vi "3. 绘制：管道分布 图.vi"(2 "放大倍数":i32, 3 "坐标原点 重新选定后 的 一维数组":dbl[](array[numeric]), 4 "color(black)输入":u32(colorbox)=8816506 caption="管道颜色") -> (0 "管道分布":picture)   [LabVIEW 2018]
panel:
  in  "初始白图":picture
  in  "fill?(F)输入":bool=TRUE caption="管道：填充？(F)"
  in  "pen输入":T1={"Width"=1, "Style"=enum."Solid"} caption="管道画笔"
  out "管道":picture
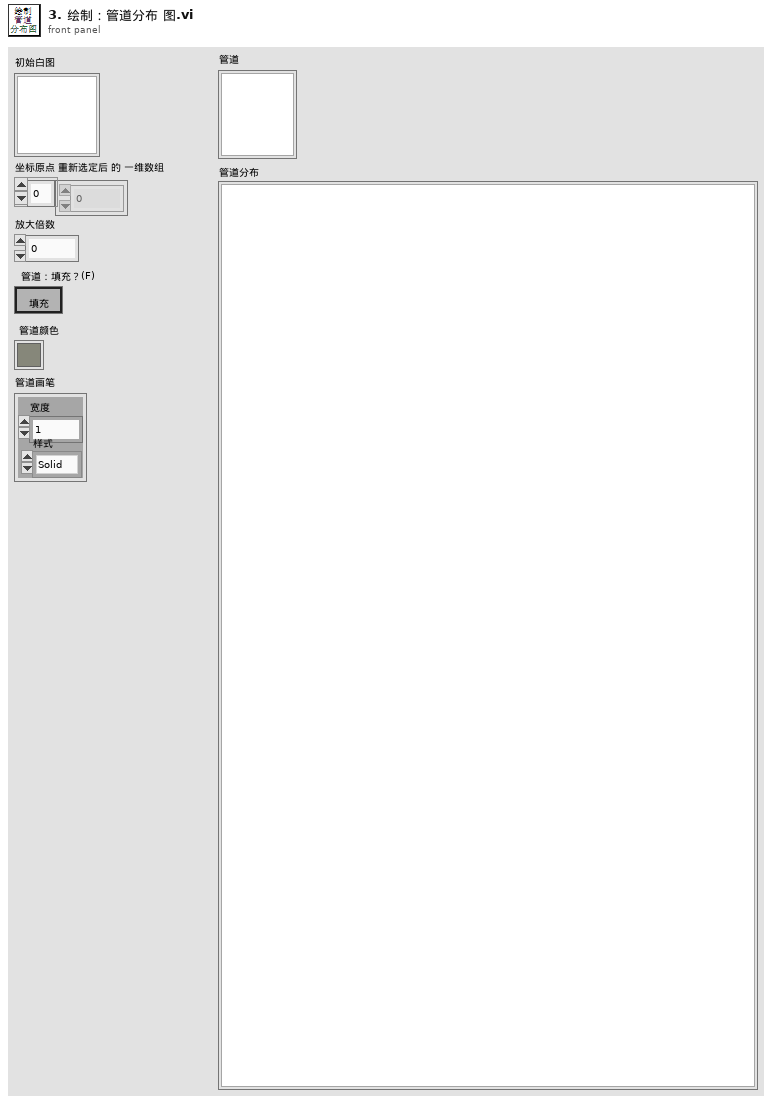
[diagram p1: front panel]
types:
  T1 = cluster{"Width":i16, "Style":enum32{"Solid", "Dash", "Dot", "DashDot", "DashDotDot"}}
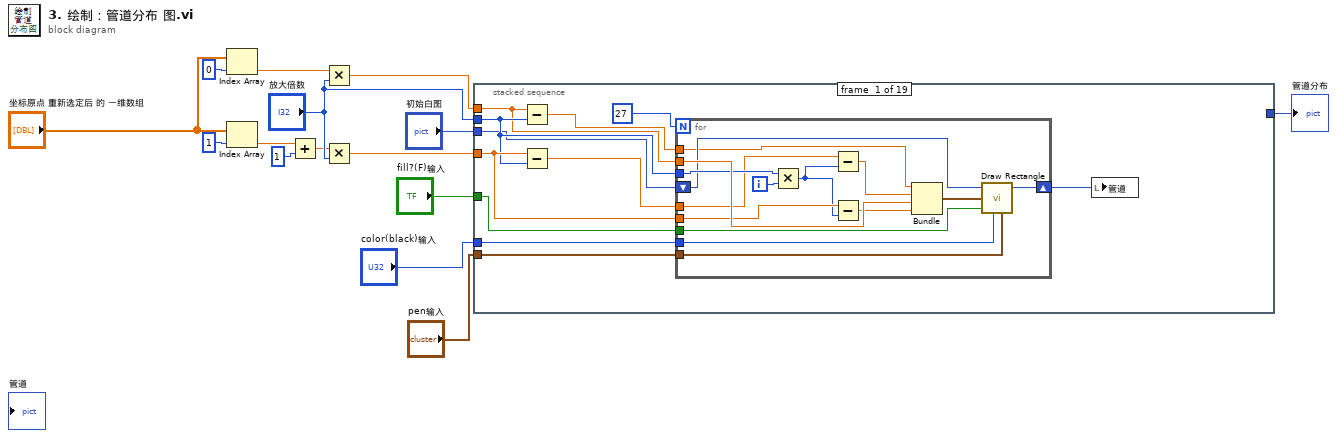
[diagram p0: block diagram]
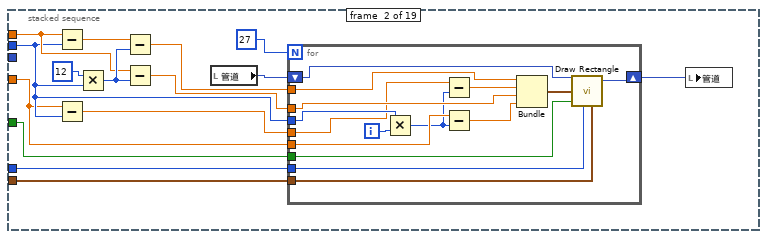
[diagram p2: hidden frame]
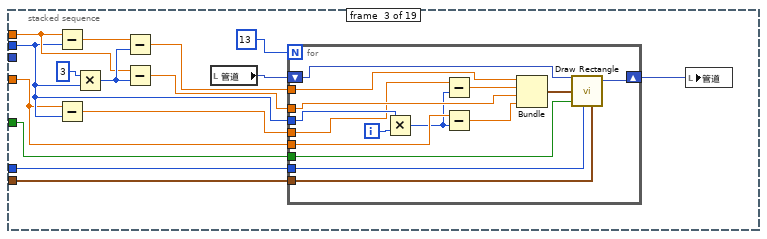
[diagram p3: hidden frame]
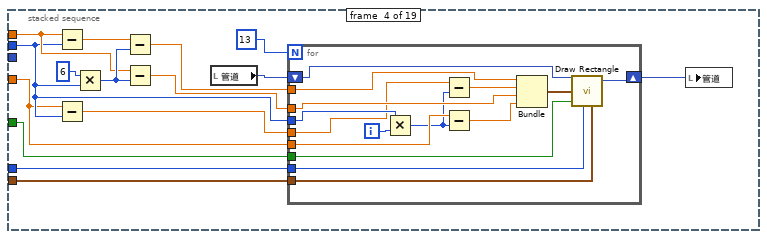
[diagram p4: hidden frame]
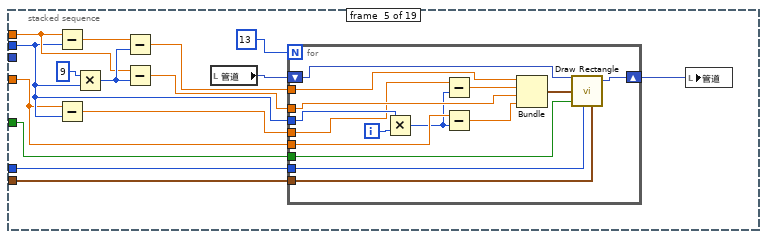
[diagram p5: hidden frame]
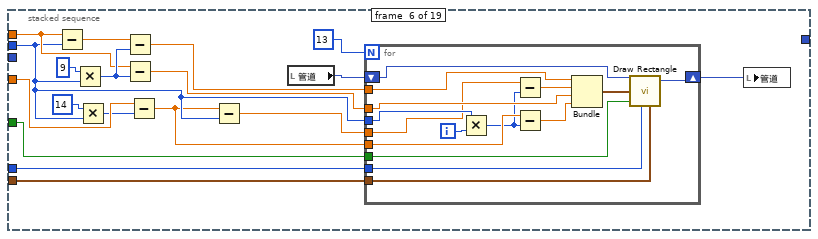
[diagram p6: hidden frame]
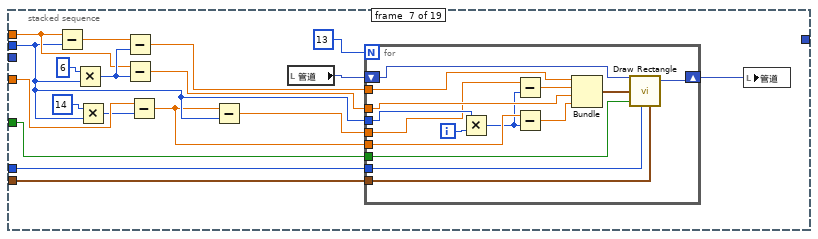
[diagram p7: hidden frame]
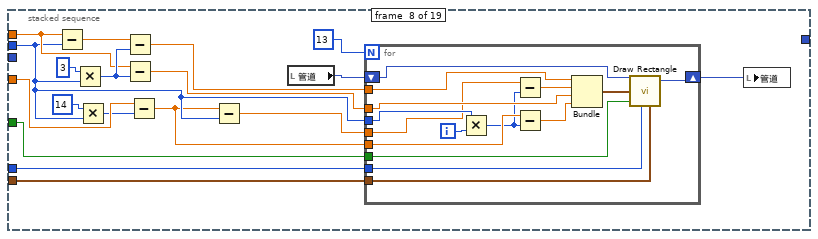
[diagram p8: hidden frame]
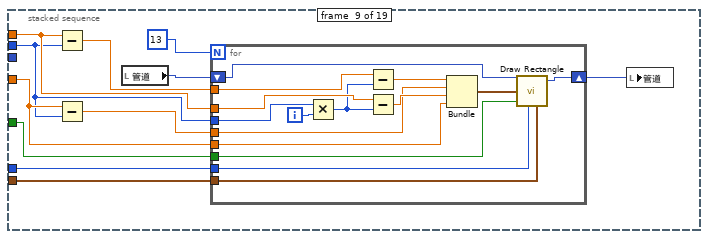
[diagram p9: hidden frame]
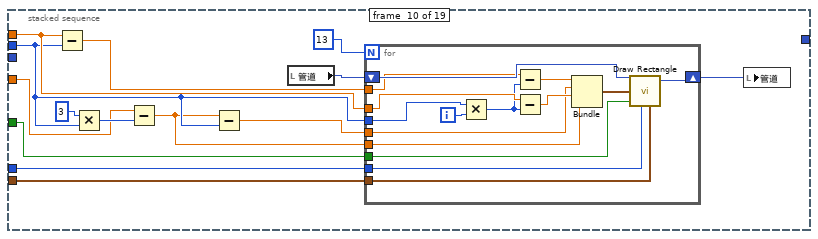
[diagram p10: hidden frame]
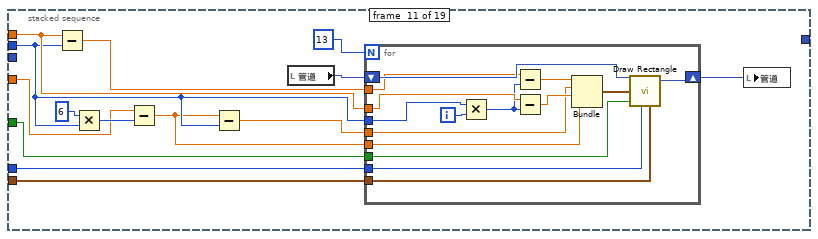
[diagram p11: hidden frame]
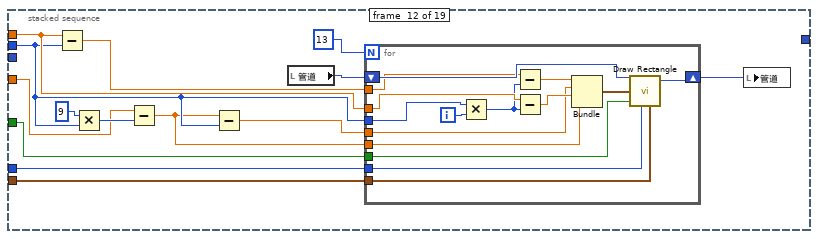
[diagram p12: hidden frame]
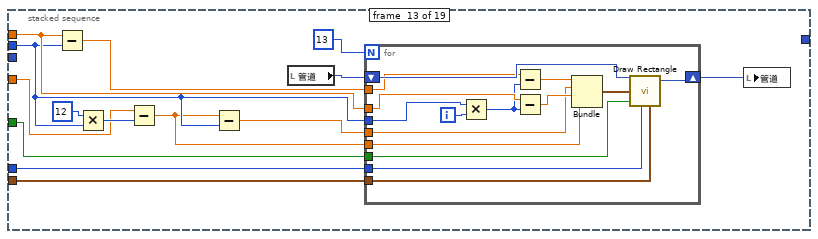
[diagram p13: hidden frame]
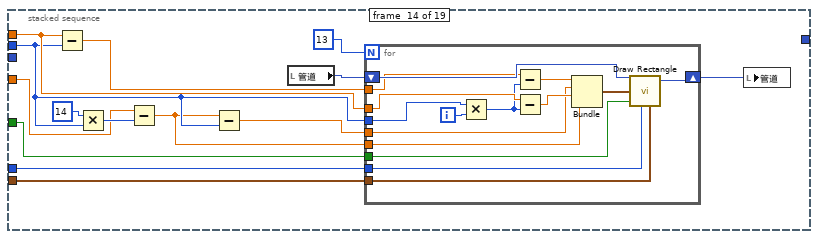
[diagram p14: hidden frame]
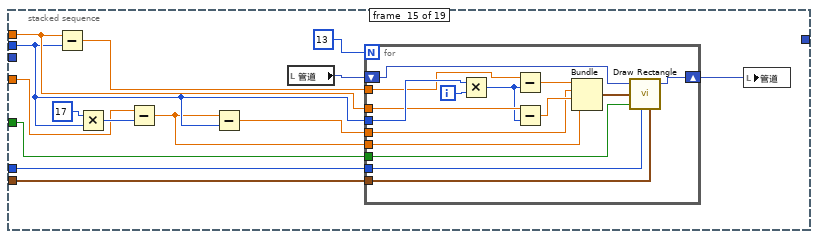
[diagram p15: hidden frame]
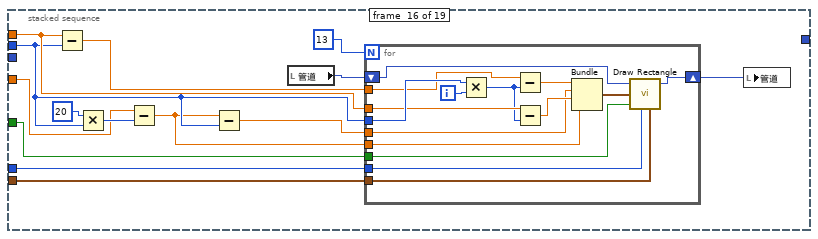
[diagram p16: hidden frame]
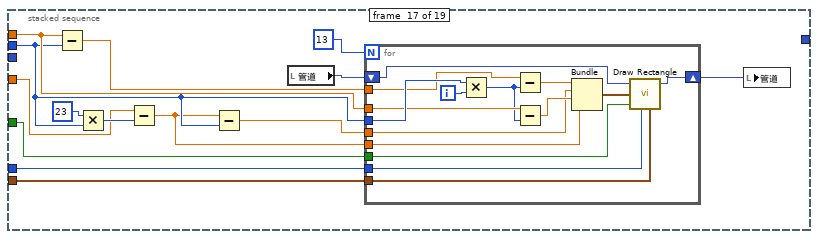
[diagram p17: hidden frame]
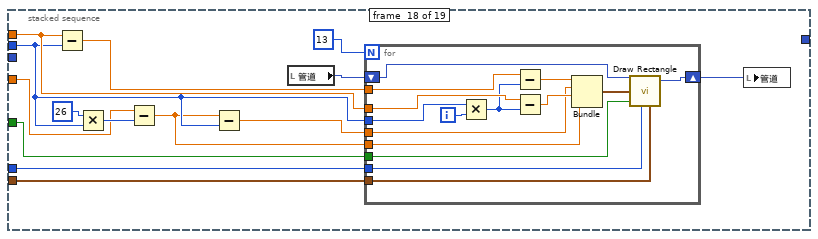
[diagram p18: hidden frame]
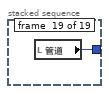
[diagram p19: hidden frame]
diagram:
  n1 = Index Array(array="坐标原点 重新选定后 的 一维数组", index=0) -> (element=w6:dbl)
  n2 = Index Array(array="坐标原点 重新选定后 的 一维数组", index=1) -> (element=w3:dbl)
  n3 = Add(x=w3, y=1) -> (x+y=w5:dbl)
  n4 = Multiply(x=w6, y="放大倍数") -> (x*y=w11:dbl)
  n5 = Multiply(x=w5, y="放大倍数") -> (x*y=w10:dbl)
  n6 = stacked-sequence {
    tunnel: "pen输入" -> [w25 w55 w85 w115 w145 w178 w211 w244 w270 w299 w328 w357 w386 w415 w444 w473 w502 w531 _]
    tunnel: "color(black)输入" -> [w24 w54 w84 w114 w144 w177 w210 w243 w269 w298 w327 w356 w385 w414 w443 w472 w501 w530 _]
    tunnel: "fill?(F)输入" -> [w23 w53 w83 w113 w143 w176 w209 w242 w268 w297 w326 w355 w384 w413 w442 w471 w500 w529 _]
    tunnel: w10 -> [w20 w44 w74 w104 w134 w165 w198 w231 w265 w290 w319 w348 w377 w406 w435 w464 w493 w522 _]
    tunnel: "放大倍数" -> [w19 w45 w75 w105 w135 w167 w200 w233 w264 w293 w322 w351 w380 w409 w438 w467 w496 w525 _]
    tunnel: w11 -> [w18 w46 w76 w106 w136 w169 w202 w235 w267 w296 w325 w354 w383 w412 w441 w470 w499 w528 _]
    tunnel: "初始白图" -> [w16 _ _ _ _ _ _ _ _ _ _ _ _ _ _ _ _ _ _]
    tunnel: [_ _ _ _ _ _ _ _ _ _ _ _ _ _ _ _ _ _ w548] -> w13
    frame #0 {
      n7 = Subtract(x=w18, y=w19) -> (x-y=w22:dbl)
      n8 = Subtract(x=w20, y=w19) -> (x-y=w21:dbl)
      n9 = for {
        N: 27 -> [_]
        shift-right: [w41] -> w17
        shift-left: w16 -> [w35]
        tunnel: w20 -> [w38]
        tunnel: w18 -> [w40]
        tunnel: w19 -> [w39]
        tunnel: w25 -> [w33]
        tunnel: w24 -> [w32]
        tunnel: w23 -> [w31]
        tunnel: w21 -> [w29]
        tunnel: w22 -> [w28]
        i -> [w30]
        n10 = Multiply(x=w39, y=w30) -> (x*y=w27:i32)
        n11 = Subtract(x=w29, y=w27) -> (x-y=w36:dbl)
        n12 = Subtract(x=w38, y=w27) -> (x-y=w37:dbl)
        n13 = Bundle(w28, w36, w40, w37) -> (w34:cluster{dbl, dbl, dbl, dbl})  [unwired: 1 in]
        n14 = call <vilib>:"Draw Rectangle.vi"("picture"=w35, "rect"=w34, "fill?(F)"=w31, "color(black)"=w32, "pen"=w33) -> ("new picture"=w41:picture)  [unwired: 4 in]
      }
      n15 = local write "管道"(w17) -> ()
    }
    frame #1 {
      n16 = Subtract(x=w46, y=w45) -> (x-y=w47:dbl)
      n17 = Subtract(x=w44, y=w45) -> (x-y=w51:dbl)
      n18 = Multiply(x=12, y=w45) -> (x*y=w48:i32)
      n19 = Subtract(x=w47, y=w48) -> (x-y=w52:dbl)
      n20 = Subtract(x=w46, y=w48) -> (x-y=w49:dbl)
      n21 = local read "管道"() -> (w42:picture)
      n22 = for {
        N: 27 -> [_]
        shift-right: [w71] -> w43
        shift-left: w42 -> [w66]
        tunnel: w44 -> [w68]
        tunnel: w49 -> [w70]
        tunnel: w45 -> [w69]
        tunnel: w55 -> [w64]
        tunnel: w54 -> [w63]
        tunnel: w53 -> [w62]
        tunnel: w51 -> [w60]
        tunnel: w52 -> [w58]
        i -> [w61]
        n23 = Multiply(x=w69, y=w61) -> (x*y=w59:i32)
        n24 = Subtract(x=w60, y=w59) -> (x-y=w57:dbl)
        n25 = Subtract(x=w68, y=w59) -> (x-y=w67:dbl)
        n26 = Bundle(w58, w57, w70, w67) -> (w65:cluster{dbl, dbl, dbl, dbl})  [unwired: 1 in]
        n27 = call <vilib>:"Draw Rectangle.vi"("picture"=w66, "rect"=w65, "fill?(F)"=w62, "color(black)"=w63, "pen"=w64) -> ("new picture"=w71:picture)  [unwired: 4 in]
      }
      n28 = local write "管道"(w43) -> ()
    }
    frame #2 {
      n29 = Subtract(x=w76, y=w75) -> (x-y=w77:dbl)
      n30 = Subtract(x=w74, y=w75) -> (x-y=w81:dbl)
      n31 = Multiply(x=3, y=w75) -> (x*y=w78:i32)
      n32 = Subtract(x=w77, y=w78) -> (x-y=w82:dbl)
      n33 = Subtract(x=w76, y=w78) -> (x-y=w79:dbl)
      n34 = local read "管道"() -> (w72:picture)
      n35 = for {
        N: 13 -> [_]
        shift-right: [w101] -> w73
        shift-left: w72 -> [w96]
        tunnel: w74 -> [w98]
        tunnel: w79 -> [w100]
        tunnel: w75 -> [w99]
        tunnel: w85 -> [w94]
        tunnel: w84 -> [w93]
        tunnel: w83 -> [w92]
        tunnel: w81 -> [w90]
        tunnel: w82 -> [w88]
        i -> [w91]
        n36 = Multiply(x=w99, y=w91) -> (x*y=w89:i32)
        n37 = Subtract(x=w90, y=w89) -> (x-y=w87:dbl)
        n38 = Subtract(x=w98, y=w89) -> (x-y=w97:dbl)
        n39 = Bundle(w88, w87, w100, w97) -> (w95:cluster{dbl, dbl, dbl, dbl})  [unwired: 1 in]
        n40 = call <vilib>:"Draw Rectangle.vi"("picture"=w96, "rect"=w95, "fill?(F)"=w92, "color(black)"=w93, "pen"=w94) -> ("new picture"=w101:picture)  [unwired: 4 in]
      }
      n41 = local write "管道"(w73) -> ()
    }
    frame #3 {
      n42 = Subtract(x=w106, y=w105) -> (x-y=w107:dbl)
      n43 = Subtract(x=w104, y=w105) -> (x-y=w111:dbl)
      n44 = Multiply(x=6, y=w105) -> (x*y=w108:i32)
      n45 = Subtract(x=w107, y=w108) -> (x-y=w112:dbl)
      n46 = Subtract(x=w106, y=w108) -> (x-y=w109:dbl)
      n47 = local read "管道"() -> (w102:picture)
      n48 = for {
        N: 13 -> [_]
        shift-right: [w131] -> w103
        shift-left: w102 -> [w126]
        tunnel: w104 -> [w128]
        tunnel: w109 -> [w130]
        tunnel: w105 -> [w129]
        tunnel: w115 -> [w124]
        tunnel: w114 -> [w123]
        tunnel: w113 -> [w122]
        tunnel: w111 -> [w120]
        tunnel: w112 -> [w118]
        i -> [w121]
        n49 = Multiply(x=w129, y=w121) -> (x*y=w119:i32)
        n50 = Subtract(x=w120, y=w119) -> (x-y=w117:dbl)
        n51 = Subtract(x=w128, y=w119) -> (x-y=w127:dbl)
        n52 = Bundle(w118, w117, w130, w127) -> (w125:cluster{dbl, dbl, dbl, dbl})  [unwired: 1 in]
        n53 = call <vilib>:"Draw Rectangle.vi"("picture"=w126, "rect"=w125, "fill?(F)"=w122, "color(black)"=w123, "pen"=w124) -> ("new picture"=w131:picture)  [unwired: 4 in]
      }
      n54 = local write "管道"(w103) -> ()
    }
    frame #4 {
      n55 = Subtract(x=w136, y=w135) -> (x-y=w137:dbl)
      n56 = Subtract(x=w134, y=w135) -> (x-y=w141:dbl)
      n57 = Multiply(x=9, y=w135) -> (x*y=w138:i32)
      n58 = Subtract(x=w137, y=w138) -> (x-y=w142:dbl)
      n59 = Subtract(x=w136, y=w138) -> (x-y=w139:dbl)
      n60 = local read "管道"() -> (w132:picture)
      n61 = for {
        N: 13 -> [_]
        shift-right: [w161] -> w133
        shift-left: w132 -> [w156]
        tunnel: w134 -> [w158]
        tunnel: w139 -> [w160]
        tunnel: w135 -> [w159]
        tunnel: w145 -> [w154]
        tunnel: w144 -> [w153]
        tunnel: w143 -> [w152]
        tunnel: w141 -> [w150]
        tunnel: w142 -> [w148]
        i -> [w151]
        n62 = Multiply(x=w159, y=w151) -> (x*y=w149:i32)
        n63 = Subtract(x=w150, y=w149) -> (x-y=w147:dbl)
        n64 = Subtract(x=w158, y=w149) -> (x-y=w157:dbl)
        n65 = Bundle(w148, w147, w160, w157) -> (w155:cluster{dbl, dbl, dbl, dbl})  [unwired: 1 in]
        n66 = call <vilib>:"Draw Rectangle.vi"("picture"=w156, "rect"=w155, "fill?(F)"=w152, "color(black)"=w153, "pen"=w154) -> ("new picture"=w161:picture)  [unwired: 4 in]
      }
      n67 = local write "管道"(w133) -> ()
    }
    frame #5 {
      n68 = Subtract(x=w169, y=w167) -> (x-y=w170:dbl)
      n69 = Multiply(x=9, y=w167) -> (x*y=w171:i32)
      n70 = Multiply(x=14, y=w167) -> (x*y=w164:i32)
      n71 = Subtract(x=w170, y=w171) -> (x-y=w175:dbl)
      n72 = Subtract(x=w169, y=w171) -> (x-y=w172:dbl)
      n73 = Subtract(x=w165, y=w164) -> (x-y=w166:dbl)
      n74 = Subtract(x=w166, y=w167) -> (x-y=w174:dbl)
      n75 = local read "管道"() -> (w162:picture)
      n76 = for {
        N: 13 -> [_]
        shift-right: [w194] -> w163
        shift-left: w162 -> [w189]
        tunnel: w166 -> [w191]
        tunnel: w172 -> [w193]
        tunnel: w167 -> [w192]
        tunnel: w178 -> [w187]
        tunnel: w177 -> [w186]
        tunnel: w176 -> [w185]
        tunnel: w174 -> [w183]
        tunnel: w175 -> [w181]
        i -> [w184]
        n77 = Multiply(x=w192, y=w184) -> (x*y=w182:i32)
        n78 = Subtract(x=w183, y=w182) -> (x-y=w180:dbl)
        n79 = Subtract(x=w191, y=w182) -> (x-y=w190:dbl)
        n80 = Bundle(w181, w180, w193, w190) -> (w188:cluster{dbl, dbl, dbl, dbl})  [unwired: 1 in]
        n81 = call <vilib>:"Draw Rectangle.vi"("picture"=w189, "rect"=w188, "fill?(F)"=w185, "color(black)"=w186, "pen"=w187) -> ("new picture"=w194:picture)  [unwired: 4 in]
      }
      n82 = local write "管道"(w163) -> ()
    }
    frame #6 {
      n83 = Subtract(x=w202, y=w200) -> (x-y=w203:dbl)
      n84 = Multiply(x=6, y=w200) -> (x*y=w204:i32)
      n85 = Multiply(x=14, y=w200) -> (x*y=w197:i32)
      n86 = Subtract(x=w203, y=w204) -> (x-y=w208:dbl)
      n87 = Subtract(x=w202, y=w204) -> (x-y=w205:dbl)
      n88 = Subtract(x=w198, y=w197) -> (x-y=w199:dbl)
      n89 = Subtract(x=w199, y=w200) -> (x-y=w207:dbl)
      n90 = local read "管道"() -> (w195:picture)
      n91 = for {
        N: 13 -> [_]
        shift-right: [w227] -> w196
        shift-left: w195 -> [w222]
        tunnel: w199 -> [w224]
        tunnel: w205 -> [w226]
        tunnel: w200 -> [w225]
        tunnel: w211 -> [w220]
        tunnel: w210 -> [w219]
        tunnel: w209 -> [w218]
        tunnel: w207 -> [w216]
        tunnel: w208 -> [w214]
        i -> [w217]
        n92 = Multiply(x=w225, y=w217) -> (x*y=w215:i32)
        n93 = Subtract(x=w216, y=w215) -> (x-y=w213:dbl)
        n94 = Subtract(x=w224, y=w215) -> (x-y=w223:dbl)
        n95 = Bundle(w214, w213, w226, w223) -> (w221:cluster{dbl, dbl, dbl, dbl})  [unwired: 1 in]
        n96 = call <vilib>:"Draw Rectangle.vi"("picture"=w222, "rect"=w221, "fill?(F)"=w218, "color(black)"=w219, "pen"=w220) -> ("new picture"=w227:picture)  [unwired: 4 in]
      }
      n97 = local write "管道"(w196) -> ()
    }
    frame #7 {
      n98 = Subtract(x=w235, y=w233) -> (x-y=w236:dbl)
      n99 = Multiply(x=3, y=w233) -> (x*y=w237:i32)
      n100 = Multiply(x=14, y=w233) -> (x*y=w230:i32)
      n101 = Subtract(x=w236, y=w237) -> (x-y=w241:dbl)
      n102 = Subtract(x=w235, y=w237) -> (x-y=w238:dbl)
      n103 = Subtract(x=w231, y=w230) -> (x-y=w232:dbl)
      n104 = Subtract(x=w232, y=w233) -> (x-y=w240:dbl)
      n105 = local read "管道"() -> (w228:picture)
      n106 = for {
        N: 13 -> [_]
        shift-right: [w260] -> w229
        shift-left: w228 -> [w255]
        tunnel: w232 -> [w257]
        tunnel: w238 -> [w259]
        tunnel: w233 -> [w258]
        tunnel: w244 -> [w253]
        tunnel: w243 -> [w252]
        tunnel: w242 -> [w251]
        tunnel: w240 -> [w249]
        tunnel: w241 -> [w247]
        i -> [w250]
        n107 = Multiply(x=w258, y=w250) -> (x*y=w248:i32)
        n108 = Subtract(x=w249, y=w248) -> (x-y=w246:dbl)
        n109 = Subtract(x=w257, y=w248) -> (x-y=w256:dbl)
        n110 = Bundle(w247, w246, w259, w256) -> (w254:cluster{dbl, dbl, dbl, dbl})  [unwired: 1 in]
        n111 = call <vilib>:"Draw Rectangle.vi"("picture"=w255, "rect"=w254, "fill?(F)"=w251, "color(black)"=w252, "pen"=w253) -> ("new picture"=w260:picture)  [unwired: 4 in]
      }
      n112 = local write "管道"(w229) -> ()
    }
    frame #8 {
      n113 = Subtract(x=w267, y=w264) -> (x-y=w266:dbl)
      n114 = Subtract(x=w265, y=w264) -> (x-y=w263:dbl)
      n115 = local read "管道"() -> (w261:picture)
      n116 = for {
        N: 13 -> [_]
        shift-right: [w286] -> w262
        shift-left: w261 -> [w285]
        tunnel: w270 -> [w283]
        tunnel: w269 -> [w282]
        tunnel: w268 -> [w281]
        tunnel: w267 -> [w278]
        tunnel: w264 -> [w279]
        tunnel: w266 -> [w274]
        tunnel: w265 -> [w276]
        tunnel: w263 -> [w275]
        i -> [w280]
        n117 = Multiply(x=w279, y=w280) -> (x*y=w273:i32)
        n118 = Subtract(x=w274, y=w273) -> (x-y=w272:dbl)
        n119 = Subtract(x=w278, y=w273) -> (x-y=w277:dbl)
        n120 = Bundle(w272, w275, w277, w276) -> (w284:cluster{dbl, dbl, dbl, dbl})  [unwired: 1 in]
        n121 = call <vilib>:"Draw Rectangle.vi"("picture"=w285, "rect"=w284, "fill?(F)"=w281, "color(black)"=w282, "pen"=w283) -> ("new picture"=w286:picture)  [unwired: 4 in]
      }
      n122 = local write "管道"(w262) -> ()
    }
    frame #9 {
      n123 = Subtract(x=w296, y=w293) -> (x-y=w295:dbl)
      n124 = Multiply(x=3, y=w293) -> (x*y=w291:i32)
      n125 = Subtract(x=w290, y=w291) -> (x-y=w289:dbl)
      n126 = Subtract(x=w289, y=w293) -> (x-y=w294:dbl)
      n127 = local read "管道"() -> (w288:picture)
      n128 = for {
        N: 13 -> [_]
        shift-right: [w315] -> w287
        shift-left: w288 -> [w314]
        tunnel: w299 -> [w312]
        tunnel: w298 -> [w311]
        tunnel: w297 -> [w310]
        tunnel: w296 -> [w307]
        tunnel: w293 -> [w308]
        tunnel: w295 -> [w303]
        tunnel: w289 -> [w305]
        tunnel: w294 -> [w304]
        i -> [w309]
        n129 = Multiply(x=w308, y=w309) -> (x*y=w302:i32)
        n130 = Subtract(x=w303, y=w302) -> (x-y=w301:dbl)
        n131 = Subtract(x=w307, y=w302) -> (x-y=w306:dbl)
        n132 = Bundle(w301, w304, w306, w305) -> (w313:cluster{dbl, dbl, dbl, dbl})  [unwired: 1 in]
        n133 = call <vilib>:"Draw Rectangle.vi"("picture"=w314, "rect"=w313, "fill?(F)"=w310, "color(black)"=w311, "pen"=w312) -> ("new picture"=w315:picture)  [unwired: 4 in]
      }
      n134 = local write "管道"(w287) -> ()
    }
    frame #10 {
      n135 = Subtract(x=w325, y=w322) -> (x-y=w324:dbl)
      n136 = Multiply(x=6, y=w322) -> (x*y=w320:i32)
      n137 = Subtract(x=w319, y=w320) -> (x-y=w318:dbl)
      n138 = Subtract(x=w318, y=w322) -> (x-y=w323:dbl)
      n139 = local read "管道"() -> (w317:picture)
      n140 = for {
        N: 13 -> [_]
        shift-right: [w344] -> w316
        shift-left: w317 -> [w343]
        tunnel: w328 -> [w341]
        tunnel: w327 -> [w340]
        tunnel: w326 -> [w339]
        tunnel: w325 -> [w336]
        tunnel: w322 -> [w337]
        tunnel: w324 -> [w332]
        tunnel: w318 -> [w334]
        tunnel: w323 -> [w333]
        i -> [w338]
        n141 = Multiply(x=w337, y=w338) -> (x*y=w331:i32)
        n142 = Subtract(x=w332, y=w331) -> (x-y=w330:dbl)
        n143 = Subtract(x=w336, y=w331) -> (x-y=w335:dbl)
        n144 = Bundle(w330, w333, w335, w334) -> (w342:cluster{dbl, dbl, dbl, dbl})  [unwired: 1 in]
        n145 = call <vilib>:"Draw Rectangle.vi"("picture"=w343, "rect"=w342, "fill?(F)"=w339, "color(black)"=w340, "pen"=w341) -> ("new picture"=w344:picture)  [unwired: 4 in]
      }
      n146 = local write "管道"(w316) -> ()
    }
    frame #11 {
      n147 = Subtract(x=w354, y=w351) -> (x-y=w353:dbl)
      n148 = Multiply(x=9, y=w351) -> (x*y=w349:i32)
      n149 = Subtract(x=w348, y=w349) -> (x-y=w347:dbl)
      n150 = Subtract(x=w347, y=w351) -> (x-y=w352:dbl)
      n151 = local read "管道"() -> (w346:picture)
      n152 = for {
        N: 13 -> [_]
        shift-right: [w373] -> w345
        shift-left: w346 -> [w372]
        tunnel: w357 -> [w370]
        tunnel: w356 -> [w369]
        tunnel: w355 -> [w368]
        tunnel: w354 -> [w365]
        tunnel: w351 -> [w366]
        tunnel: w353 -> [w361]
        tunnel: w347 -> [w363]
        tunnel: w352 -> [w362]
        i -> [w367]
        n153 = Multiply(x=w366, y=w367) -> (x*y=w360:i32)
        n154 = Subtract(x=w361, y=w360) -> (x-y=w359:dbl)
        n155 = Subtract(x=w365, y=w360) -> (x-y=w364:dbl)
        n156 = Bundle(w359, w362, w364, w363) -> (w371:cluster{dbl, dbl, dbl, dbl})  [unwired: 1 in]
        n157 = call <vilib>:"Draw Rectangle.vi"("picture"=w372, "rect"=w371, "fill?(F)"=w368, "color(black)"=w369, "pen"=w370) -> ("new picture"=w373:picture)  [unwired: 4 in]
      }
      n158 = local write "管道"(w345) -> ()
    }
    frame #12 {
      n159 = Subtract(x=w383, y=w380) -> (x-y=w382:dbl)
      n160 = Multiply(x=12, y=w380) -> (x*y=w378:i32)
      n161 = Subtract(x=w377, y=w378) -> (x-y=w376:dbl)
      n162 = Subtract(x=w376, y=w380) -> (x-y=w381:dbl)
      n163 = local read "管道"() -> (w375:picture)
      n164 = for {
        N: 13 -> [_]
        shift-right: [w402] -> w374
        shift-left: w375 -> [w401]
        tunnel: w386 -> [w399]
        tunnel: w385 -> [w398]
        tunnel: w384 -> [w397]
        tunnel: w383 -> [w394]
        tunnel: w380 -> [w395]
        tunnel: w382 -> [w390]
        tunnel: w376 -> [w392]
        tunnel: w381 -> [w391]
        i -> [w396]
        n165 = Multiply(x=w395, y=w396) -> (x*y=w389:i32)
        n166 = Subtract(x=w390, y=w389) -> (x-y=w388:dbl)
        n167 = Subtract(x=w394, y=w389) -> (x-y=w393:dbl)
        n168 = Bundle(w388, w391, w393, w392) -> (w400:cluster{dbl, dbl, dbl, dbl})  [unwired: 1 in]
        n169 = call <vilib>:"Draw Rectangle.vi"("picture"=w401, "rect"=w400, "fill?(F)"=w397, "color(black)"=w398, "pen"=w399) -> ("new picture"=w402:picture)  [unwired: 4 in]
      }
      n170 = local write "管道"(w374) -> ()
    }
    frame #13 {
      n171 = Subtract(x=w412, y=w409) -> (x-y=w411:dbl)
      n172 = Multiply(x=14, y=w409) -> (x*y=w407:i32)
      n173 = Subtract(x=w406, y=w407) -> (x-y=w405:dbl)
      n174 = Subtract(x=w405, y=w409) -> (x-y=w410:dbl)
      n175 = local read "管道"() -> (w404:picture)
      n176 = for {
        N: 13 -> [_]
        shift-right: [w431] -> w403
        shift-left: w404 -> [w430]
        tunnel: w415 -> [w428]
        tunnel: w414 -> [w427]
        tunnel: w413 -> [w426]
        tunnel: w412 -> [w423]
        tunnel: w409 -> [w424]
        tunnel: w411 -> [w419]
        tunnel: w405 -> [w421]
        tunnel: w410 -> [w420]
        i -> [w425]
        n177 = Multiply(x=w424, y=w425) -> (x*y=w418:i32)
        n178 = Subtract(x=w419, y=w418) -> (x-y=w417:dbl)
        n179 = Subtract(x=w423, y=w418) -> (x-y=w422:dbl)
        n180 = Bundle(w417, w420, w422, w421) -> (w429:cluster{dbl, dbl, dbl, dbl})  [unwired: 1 in]
        n181 = call <vilib>:"Draw Rectangle.vi"("picture"=w430, "rect"=w429, "fill?(F)"=w426, "color(black)"=w427, "pen"=w428) -> ("new picture"=w431:picture)  [unwired: 4 in]
      }
      n182 = local write "管道"(w403) -> ()
    }
    frame #14 {
      n183 = Subtract(x=w441, y=w438) -> (x-y=w440:dbl)
      n184 = Multiply(x=17, y=w438) -> (x*y=w436:i32)
      n185 = Subtract(x=w435, y=w436) -> (x-y=w434:dbl)
      n186 = Subtract(x=w434, y=w438) -> (x-y=w439:dbl)
      n187 = local read "管道"() -> (w433:picture)
      n188 = for {
        N: 13 -> [_]
        shift-right: [w460] -> w432
        shift-left: w433 -> [w459]
        tunnel: w444 -> [w457]
        tunnel: w443 -> [w456]
        tunnel: w442 -> [w455]
        tunnel: w441 -> [w452]
        tunnel: w438 -> [w453]
        tunnel: w440 -> [w448]
        tunnel: w434 -> [w450]
        tunnel: w439 -> [w449]
        i -> [w454]
        n189 = Multiply(x=w453, y=w454) -> (x*y=w447:i32)
        n190 = Subtract(x=w448, y=w447) -> (x-y=w446:dbl)
        n191 = Subtract(x=w452, y=w447) -> (x-y=w451:dbl)
        n192 = Bundle(w446, w449, w451, w450) -> (w458:cluster{dbl, dbl, dbl, dbl})  [unwired: 1 in]
        n193 = call <vilib>:"Draw Rectangle.vi"("picture"=w459, "rect"=w458, "fill?(F)"=w455, "color(black)"=w456, "pen"=w457) -> ("new picture"=w460:picture)  [unwired: 4 in]
      }
      n194 = local write "管道"(w432) -> ()
    }
    frame #15 {
      n195 = Subtract(x=w470, y=w467) -> (x-y=w469:dbl)
      n196 = Multiply(x=20, y=w467) -> (x*y=w465:i32)
      n197 = Subtract(x=w464, y=w465) -> (x-y=w463:dbl)
      n198 = Subtract(x=w463, y=w467) -> (x-y=w468:dbl)
      n199 = local read "管道"() -> (w462:picture)
      n200 = for {
        N: 13 -> [_]
        shift-right: [w489] -> w461
        shift-left: w462 -> [w488]
        tunnel: w473 -> [w486]
        tunnel: w472 -> [w485]
        tunnel: w471 -> [w484]
        tunnel: w470 -> [w481]
        tunnel: w467 -> [w482]
        tunnel: w469 -> [w477]
        tunnel: w463 -> [w479]
        tunnel: w468 -> [w478]
        i -> [w483]
        n201 = Multiply(x=w482, y=w483) -> (x*y=w476:i32)
        n202 = Subtract(x=w477, y=w476) -> (x-y=w475:dbl)
        n203 = Subtract(x=w481, y=w476) -> (x-y=w480:dbl)
        n204 = Bundle(w475, w478, w480, w479) -> (w487:cluster{dbl, dbl, dbl, dbl})  [unwired: 1 in]
        n205 = call <vilib>:"Draw Rectangle.vi"("picture"=w488, "rect"=w487, "fill?(F)"=w484, "color(black)"=w485, "pen"=w486) -> ("new picture"=w489:picture)  [unwired: 4 in]
      }
      n206 = local write "管道"(w461) -> ()
    }
    frame #16 {
      n207 = Subtract(x=w499, y=w496) -> (x-y=w498:dbl)
      n208 = Multiply(x=23, y=w496) -> (x*y=w494:i32)
      n209 = Subtract(x=w493, y=w494) -> (x-y=w492:dbl)
      n210 = Subtract(x=w492, y=w496) -> (x-y=w497:dbl)
      n211 = local read "管道"() -> (w490:picture)
      n212 = for {
        N: 13 -> [_]
        shift-right: [w518] -> w491
        shift-left: w490 -> [w517]
        tunnel: w502 -> [w515]
        tunnel: w501 -> [w514]
        tunnel: w500 -> [w513]
        tunnel: w499 -> [w510]
        tunnel: w496 -> [w511]
        tunnel: w498 -> [w506]
        tunnel: w492 -> [w508]
        tunnel: w497 -> [w507]
        i -> [w512]
        n213 = Multiply(x=w511, y=w512) -> (x*y=w505:i32)
        n214 = Subtract(x=w506, y=w505) -> (x-y=w504:dbl)
        n215 = Subtract(x=w510, y=w505) -> (x-y=w509:dbl)
        n216 = Bundle(w504, w507, w509, w508) -> (w516:cluster{dbl, dbl, dbl, dbl})  [unwired: 1 in]
        n217 = call <vilib>:"Draw Rectangle.vi"("picture"=w517, "rect"=w516, "fill?(F)"=w513, "color(black)"=w514, "pen"=w515) -> ("new picture"=w518:picture)  [unwired: 4 in]
      }
      n218 = local write "管道"(w491) -> ()
    }
    frame #17 {
      n219 = Subtract(x=w528, y=w525) -> (x-y=w527:dbl)
      n220 = Multiply(x=26, y=w525) -> (x*y=w523:i32)
      n221 = Subtract(x=w522, y=w523) -> (x-y=w521:dbl)
      n222 = Subtract(x=w521, y=w525) -> (x-y=w526:dbl)
      n223 = local read "管道"() -> (w519:picture)
      n224 = for {
        N: 13 -> [_]
        shift-right: [w547] -> w520
        shift-left: w519 -> [w546]
        tunnel: w531 -> [w544]
        tunnel: w530 -> [w543]
        tunnel: w529 -> [w542]
        tunnel: w528 -> [w539]
        tunnel: w525 -> [w540]
        tunnel: w527 -> [w535]
        tunnel: w521 -> [w537]
        tunnel: w526 -> [w536]
        i -> [w541]
        n225 = Multiply(x=w540, y=w541) -> (x*y=w534:i32)
        n226 = Subtract(x=w535, y=w534) -> (x-y=w533:dbl)
        n227 = Subtract(x=w539, y=w534) -> (x-y=w538:dbl)
        n228 = Bundle(w533, w536, w538, w537) -> (w545:cluster{dbl, dbl, dbl, dbl})  [unwired: 1 in]
        n229 = call <vilib>:"Draw Rectangle.vi"("picture"=w546, "rect"=w545, "fill?(F)"=w542, "color(black)"=w543, "pen"=w544) -> ("new picture"=w547:picture)  [unwired: 4 in]
      }
      n230 = local write "管道"(w520) -> ()
    }
    frame #18 {
      n231 = local read "管道"() -> (w548:picture)
    }
  }
  "管道分布" <- w13
